vi "Add Two Analog Inputs.vi"() -> ()   [LabVIEW 2018]
uses:
  <vilib>/rvi/Emulation/niFpgaGetClockAttributes.vi
  <vilib>/rvi/Emulation/niFpgaSctlEmulationGetInTimedLoop.vi
  <vilib>/rvi/Emulation/niFpgaEmulationReportErrorSimple.vi
  <vilib>/rvi/eio/common/nirviEmuTemplateMethod_errors.vi
  <vilib>/rvi/Emulation/niFpgaCriticalErrorInLSC.vi
  <vilib>/eio/EIONode/EIONode.xnode
panel:
  in  "Count(Ticks)":u32
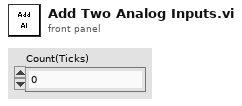
[diagram p1: front panel]
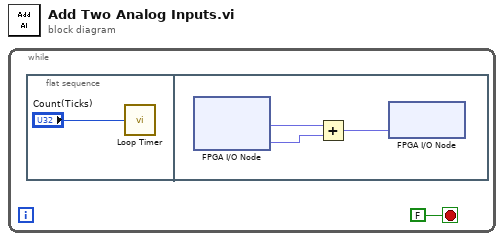
[diagram p0: block diagram]
diagram:
  n1 = while {
    stop <- FALSE stop-if-true
    n2 = flat-sequence {
      frame #0 {
        n3 = call "Loop Timer"("Count(Ticks)"="Count(Ticks)") -> ()  [unwired: 1 out]
      }
      frame #1 {
        n4 = xnode "FPGA I/O Node"() -> ("AI0"=w5:fxp<+/-,24,5>, "AI1"=w4:fxp<+/-,24,5>)  [unwired: 2 in, 2 out]
        n5 = Add(x=w5, y=w4) -> (x+y=w3:fxp<+/-,25,6>)
        n6 = xnode "FPGA I/O Node"("AO0"=w3) -> ()  [unwired: 1 in, 1 out]
      }
    }
  }
